vi "Update Project Organization.vi"(8 "error in (no error)":errorcluster, 10 "ProjectOrganization":T1, 11 "BuildServer in":refnum<class "BuildServer.lvclass">) -> (0 "error out":errorcluster, 3 "BuildServer out":refnum<class "BuildServer.lvclass">)   [LabVIEW 2017, in "BuildServer.lvlib" / "BuildServer.lvclass"]
uses:
  BuildServer.lvclass
  C:/Program Files (x86)/National Instruments/LabVIEW 2017/vi.lib/ActorFramework/Actor/Actor.lvclass
  ProjectOrganization.ctl
  BuildServer.lvclass/BuildServer.ctl
  <vilib>/ActorFramework/Actor/Actor.lvclass/Actor.ctl
  <vilib>/ActorFramework/Message Enqueuer/Message Enqueuer.lvclass/Message Enqueuer.ctl
  <vilib>/ActorFramework/Message Enqueuer/Init from Existing Queue.vi
  <vilib>/ActorFramework/Message Enqueuer/Enqueue.vi
  BuildServer Messages/Update Tree Msg/Update Tree Msg.lvclass
  C:/Program Files (x86)/National Instruments/LabVIEW 2017/vi.lib/ActorFramework/Message/Message.lvclass
  <vilib>/ActorFramework/Message Priority Queue/Priority Enqueue.vi
  <vilib>/ActorFramework/Message Enqueuer/Message Enqueuer.lvclass
  <vilib>/ActorFramework/Actor/Actor.lvclass
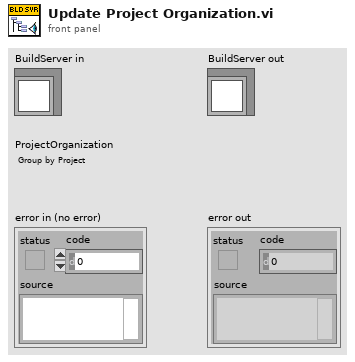
[diagram p1: front panel]
types:
  T1 = typedef "BuildServer.lvlib/BuildServer.lvclass/ProjectOrganization.ctl" = enum16{"Group by Project", "Group by Target", "Group by Type", "Group by Name"}
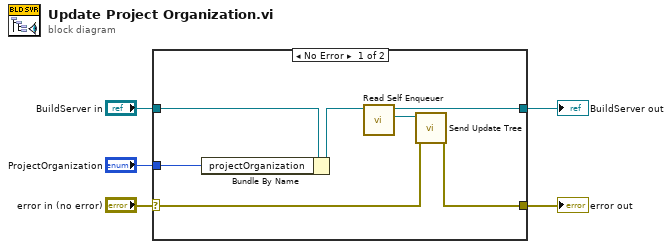
[diagram p0: block diagram]
diagram:
  n1 = case shown="No Error" "error in (no error)" {
    selector: "error in (no error)" -> [w7 w13]
    tunnel: [w6 w13] -> w4
    tunnel: [w9 w12] -> w2
    tunnel: "BuildServer in" -> [w11 w12]
    tunnel: "ProjectOrganization" -> [w10 _]
    frame No Error {
      n2 = Bundle By Name(cluster=w11, "projectOrganization"=w10) -> (w9:refnum<class "BuildServer.lvclass">)
      n3 = call <vilib>:"Read Self Enqueuer.vi"("Actor"=w9) -> ("Self Enqueuer"=w8:refnum<class "Message Enqueuer.lvclass">)  [unwired: 10 in]
      n4 = call "Send Update Tree.vi"("error in (no error)"=w7, "Message Enqueuer in"=w8) -> ("error out"=w6:errorcluster)  [unwired: 8 in, 1 out]
    }
    frame Error {
    }
  }
  "error out" <- w4
  "BuildServer out" <- w2
